vi "Decode Error Listbox.vi"(8 "error in (no error)":errorcluster, 11 "Data":variant) -> (0 "error out":errorcluster, 3 "Data out":variant)   [LabVIEW 2026, in "TALOS.lvlib" / "Guardian.lvlib" / "Guardian.lvclass"]
uses:
  Guardian.lvclass
  Internal uServices/System uServices/Common GUI v3/Common GUI v3/Error Listbox Msg.ctl
  Internal uServices/System uServices/Common GUI v3/Common GUI v3/Error Listbox Msg Action.ctl
  Internal uServices/System uServices/Error Manager/Error Info.ctl
  Internal uServices/System uServices/Error Manager/Error Manager.lvclass
  Internal uServices/System uServices/Common GUI v3/Common GUI v3/Common GUI v3.lvclass
  TALOS.lvlib
  <vilib>/MultiError/TokenizeJSON/Multi Error Cluster.lvlib
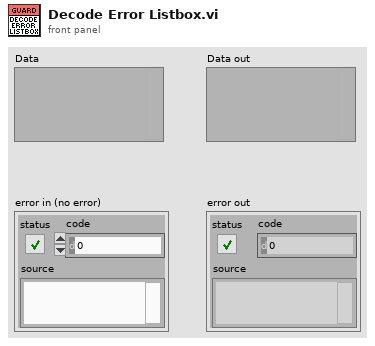
[diagram p1: front panel]
types:
  T1 = typedef "TALOS.lvlib/Common GUI v3.lvlib/Common GUI v3.lvclass/Error Listbox Msg Action.ctl" = enum16{"Add", "Remove", "Clear"}
  T2 = typedef "TALOS.lvlib/Common GUI v3.lvlib/Common GUI v3.lvclass/Error Listbox Msg.ctl" = cluster{"Action":T1, "Error Info":T3}
  T3 = typedef "TALOS.lvlib/Error Manager.lvlib/Error Manager.lvclass/Error Info.ctl" = cluster{"error out":errorcluster, "Time Stamp":timestamp, "Machine Name":string, "GUID":string}
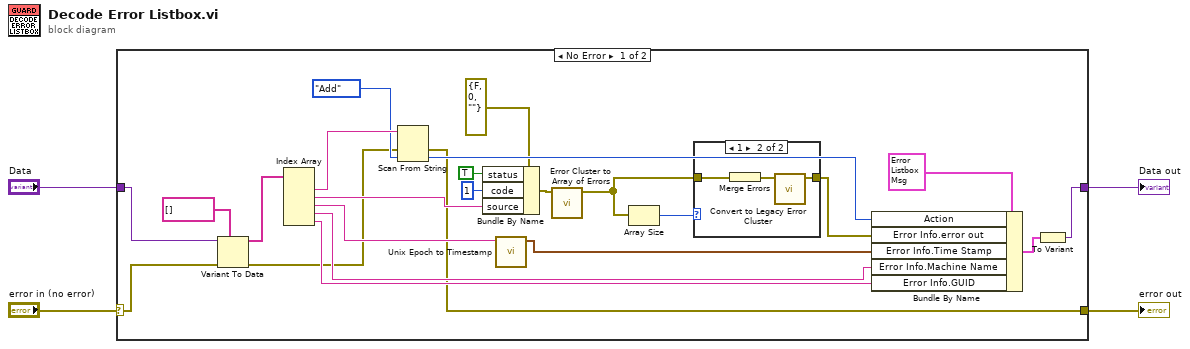
[diagram p0: block diagram]
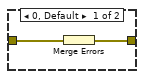
[diagram p2: hidden frame]
diagram:
  n1 = case shown="No Error" "error in (no error)" {
    selector: "error in (no error)" -> [w6 w34]
    tunnel: "Data" -> [w5 w35]
    tunnel: [w14 w35] -> w2
    tunnel: [w13 w34] -> w1
    frame No Error {
      n2 = Variant To Data(error in=w6, type=string[] [], Variant=w5) -> (data=w12:string[], error out=w8:errorcluster)
      n3 = Index Array(array=w12) -> (element #1=w28:string, element #2=w16:string, element #3=w23:string, element #4=w24:string, element #5=w25:string)  [unwired: 5 in]
      n4 = Scan From String(input string=w28, error in=w8, default 1=Error_Listbox_Msg_Action."Add" ("Action")) -> (error out=w13:errorcluster, output 1=w21:T1)  [unwired: 2 in, 2 out]
      n5 = Bundle By Name(cluster=errorcluster {"status"=FALSE, "code"=0, "source"=""} ("error constant"), "status"=TRUE, "code"=1, "source"=w16) -> (w17:errorcluster)
      n6 = call "Unix Epoch to Timestamp.vi"("String"=w23) -> ("Time Stamp"=w22:timestamp)  [unwired: 10 in]
      n7 = call <vilib>:"Error Cluster to Array of Errors.vi"("error"=w17) -> ("array of errors"=w10:errorcluster[])  [unwired: 10 in]
      n8 = Array Size(array=w10) -> (size(s)=w11:i32)
      n9 = case shown="1" w11 {
        tunnel: [w29 w31] -> w9
        tunnel: w10 -> [w30 w32]
        frame 0, Default {
          n10 = Merge Errors(w30) -> (w29:errorcluster)
        }
        frame 1 {
          n11 = Merge Errors(w32) -> (w33:errorcluster)
          n12 = call <vilib>:"Convert to Legacy Error Cluster.vi"("error in"=w33) -> ("error out"=w31:errorcluster)  [unwired: 10 in]
        }
      }
      n13 = Bundle By Name(cluster=T2 {"Action"=enum."Add", "Error Info"={"error out"={"status"=FALSE, "code"=0, "source"=""}, "Time Stamp"=timestamp(0 s since 1904-01-01), "Machine Name"="", "GUID"=""}} ("Error Listbox Msg"), "Action"=w21, "Error Info.error out"=w9, "Error Info.Time Stamp"=w22, "Error Info.Machine Name"=w24, "Error Info.GUID"=w25) -> (w15:T2)
      n14 = To Variant(anything=w15) -> (Variant=w14:variant)
    }
    frame Error {
    }
  }
  "error out" <- w1
  "Data out" <- w2
